vi "时间计算.vi"(10 "数组":string[][](array[string]), 11 "循环次数":i32) -> (3 "x*y":dbl)   [LabVIEW 2021]
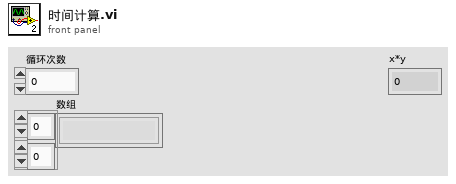
[diagram p1: front panel]
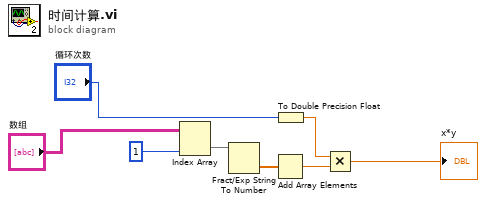
[diagram p0: block diagram]
diagram:
  n1 = Index Array(array="数组", index (col)=1 ("禁用的索引 (列)")) -> (element=w7:string[])  [unwired: 1 in]
  n2 = Fract/Exp String To Number(string=w7) -> (number=w6:dbl[])  [unwired: 3 in, 1 out]
  n3 = Add Array Elements(numeric array=w6) -> (sum=w5:dbl)
  n4 = To Double Precision Float(number="循环次数") -> (double precision float=w4:dbl)
  n5 = Multiply(x=w4, y=w5) -> (x*y=→"x*y":dbl)
